vi "Configure Range Table (Spurious Emissions - Peak).vi"(0 "VISA resource name":refnum<visa-resource-name>, 5 "Peak Excursion List":dbl[](array[numeric])=[6.0, 6.0] format="%#.6g", 9 "Peak Threshold List":dbl[](array[numeric])=[-90.0, -90.0] format="%#.6g", 11 "error in (no error)":errorcluster) -> (4 "VISA resource name out":refnum<visa-resource-name>, 15 "error out":errorcluster)   [LabVIEW 2014, in "Agilent MXA Series.lvlib"]
doc: "Configures the Peak settings under Range Table for Spurious Emissions measurement type."
uses:
  Agilent MXA Series.lvlib
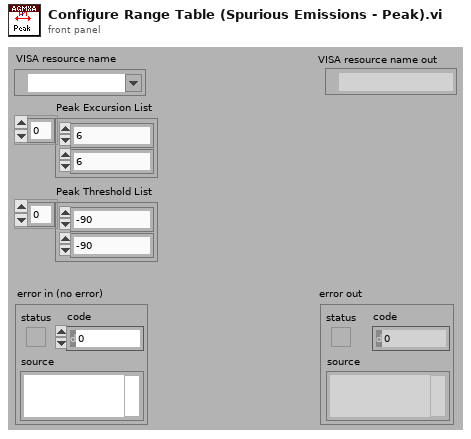
[diagram p1: front panel]
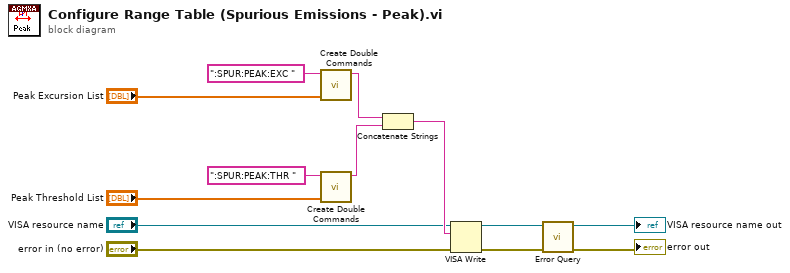
[diagram p0: block diagram]
diagram:
  n1 = call "Create Double Commands.vi"("Double Values"="Peak Excursion List", "Commands"=":SPUR:PEAK:EXC ") -> ("Result"=w9:string)  [unwired: 9 in]
  n2 = call "Create Double Commands.vi"("Double Values"="Peak Threshold List", "Commands"=":SPUR:PEAK:THR ") -> ("Result"=w8:string)  [unwired: 9 in]
  n3 = Concatenate Strings(w9, w8) -> (w5:string)
  n4 = VISA Write(VISA resource name="VISA resource name", write buffer=w5, error in (no error)="error in (no error)") -> (VISA resource name out=w6:refnum<visa-resource-name>, error out=w7:errorcluster)  [unwired: 1 out]
  n5 = call "Error Query.vi"("error in (no error)"=w7, "VISA resource name"=w6) -> ("error out"=→"error out":errorcluster, "VISA resource name out"=→"VISA resource name out":refnum<visa-resource-name>)  [unwired: 6 in, 2 out]
